vi "Get Force Reading.vi"(8 "error in (no error)":errorcluster, 11 "ESM303 in":refnum<class "ESM303.lvclass">) -> (0 "error out":errorcluster, 2 "Reading":dbl format="%.4f", 3 "ESM303 out":refnum<class "ESM303.lvclass">)   [LabVIEW 2018, in "ESM303.lvlib" / "ESM303.lvclass"]
uses:
  ESM303.lvclass
  builds/Force Test Stand/Force Test Stand/Force Test Stand.lvlibp/Force Test Stand.lvclass
  C:/Projects/LabVIEW/In-Progress/Jose Rivero-Diaz/builds/Force Test Stand/Force Test Stand/Force Test Stand.lvlibp/Force Test Stand.lvclass
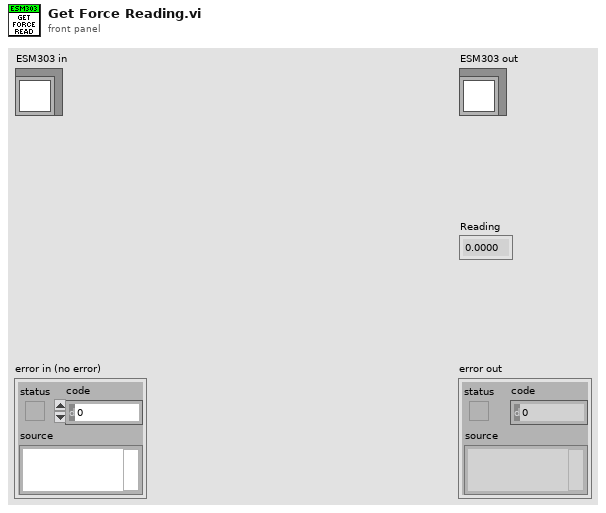
[diagram p1: front panel]
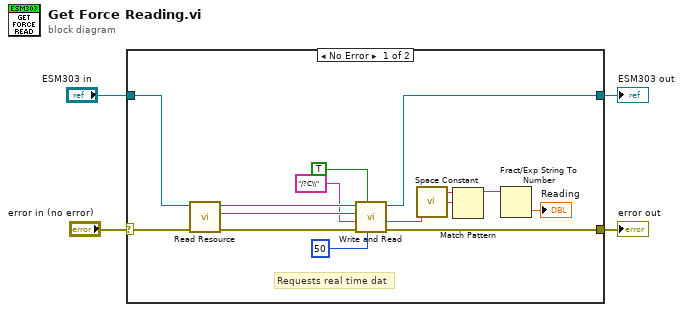
[diagram p0: block diagram]
diagram:
  n1 = case shown="No Error" "error in (no error)" {
    selector: "error in (no error)" -> [w18 w20]
    tunnel: [w10 w20] -> w3
    tunnel: [w9 w19] -> w2
    tunnel: "ESM303 in" -> [w17 w19]
    frame No Error {
      # "Requests real time dat"
      n2 = call "Read Resource.vi"("error in (no error)"=w18, "Force Test Stand in"=w17) -> ("error out"=w14:errorcluster, "Resource"=w15:refnum<visa-resource-name>, "Force Test Stand out"=w16:refnum<class "ESM303.lvclass">)  [unwired: 7 in]
      n3 = call "Write and Read.vi"("Delay Before Read (ms)"=50, "Write & Read"=TRUE, "error in (no error)"=w14, "Command"="/?C\\", "VISA Refnum in"=w15, "ESM303 in"=w16) -> ("error out"=w10:errorcluster, "Response"=w6:string, "ESM303 out"=w9:refnum<class "ESM303.lvclass">)  [unwired: 3 in]
      n4 = call <vilib>:"Space Constant.vi"() -> ("String"=w7:string)
      n5 = Match Pattern(string=w6, regular expression=w7) -> (before substring=w5:string)  [unwired: 1 in, 3 out]
      n6 = Fract/Exp String To Number(string=w5) -> (number=→"Reading":dbl)  [unwired: 3 in, 1 out]
    }
    frame Error {
    }
  }
  "error out" <- w3
  "ESM303 out" <- w2
